vi "LCC Write Set Point.vi"(8 "error in (no error)":errorcluster caption="Fehler (Eingang, kein Fehler)", 10 "Setpoint":dbl, 11 "Channel Handle":i64) -> (0 "error out":errorcluster caption="Fehler (Ausgang)")   [LabVIEW 2021, in "labbCAN_Controller_API.lvlib"]
doc: "LCC_Func long LCC_CALL LCC_WriteSetPoint(dev_hdl ChanHdl, double fSetPointValue);"
uses:
  labbCAN_Controller_API.lvlib
  labbCAN_Controller_API.dll
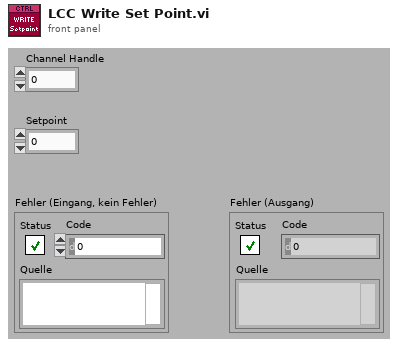
[diagram p1: front panel]
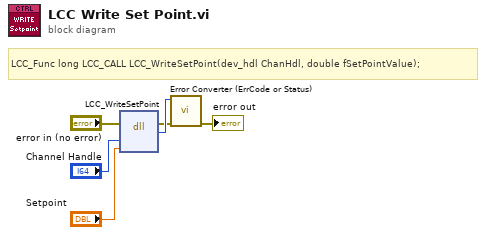
[diagram p0: block diagram]
diagram:
  # "LCC_Func long LCC_CALL LCC_WriteSetPoint(dev_hdl ChanHdl, double fSetPointValue);"
  n1 = dll-call lib="C:/Users/olaja/AppData/Local/CETONI_SDK/labbCAN_Controller_API.*" fn="LCC_WriteSetPoint"(error in="error in (no error)", "ChanHdl"="Channel Handle", "fSetPointValue"="Setpoint") -> (error out=w2:errorcluster, "Rückgabetyp"=w3:i32)  [unwired: 4 in, 1 out]
  n2 = call "Error Converter (ErrCode or Status).vi"("error in (no error)"=w2, "error code"=w3) -> ("error out"=→"error out":errorcluster)  [unwired: 9 in]
